vi "configure.vi"(8 "error in (no error)":errorcluster, 9 "Value":i32, 10 "ILC":refnum<class "ILC.lvclass">, 11 "ConfigureILCSSRStrategy in":refnum<class "ConfigureILCSSRStrategy.lvclass">) -> (0 "error out":errorcluster, 3 "ConfigureILCSSRStrategy out":refnum<class "ConfigureILCSSRStrategy.lvclass">)   [LabVIEW 2015, in "ConfigureILCSSRStrategy.lvclass"]
uses:
  ConfigureILCSSRStrategy.lvclass
  <userlib>/Common/ilc/ILC/ILC.lvclass
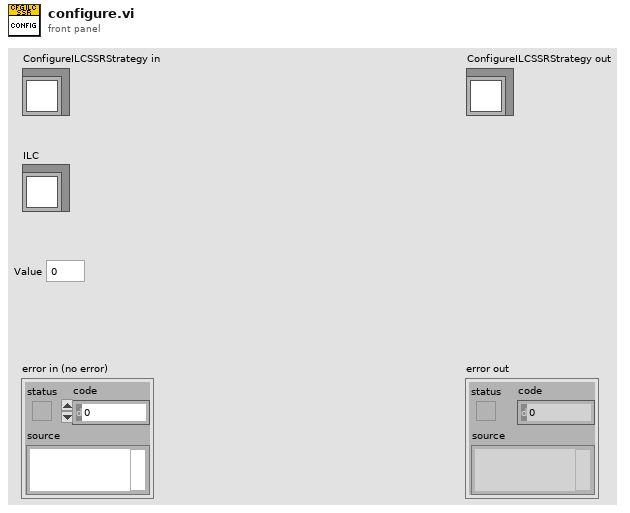
[diagram p1: front panel]
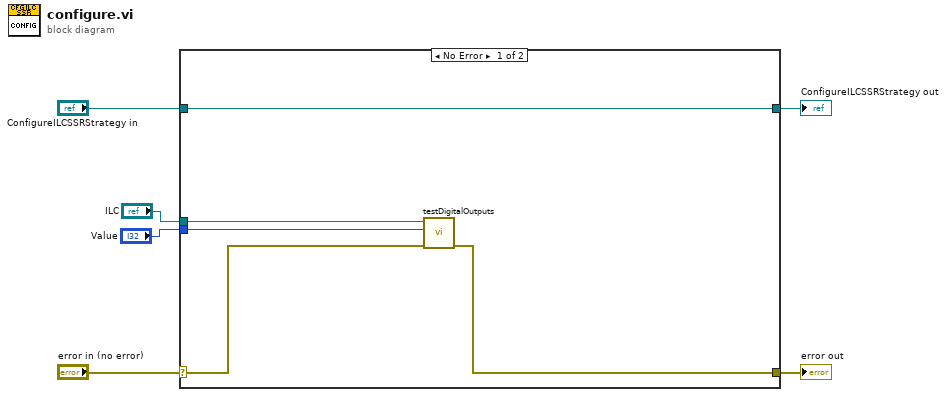
[diagram p0: block diagram]
diagram:
  n1 = case shown="No Error" "error in (no error)" {
    selector: "error in (no error)" -> [w7 w13]
    tunnel: [w8 w13] -> w5
    tunnel: [w11 w12] -> w3
    tunnel: "ConfigureILCSSRStrategy in" -> [w11 w12]
    tunnel: "ILC" -> [w10 _]
    tunnel: "Value" -> [w9 _]
    frame No Error {
      n2 = call <userlib>:"testDigitalOutputs.vi"("error in (no error)"=w7, "Digital Output Value"=w9, "ILC in"=w10) -> ("error out"=w8:errorcluster)  [unwired: 7 in, 1 out]
    }
    frame Error {
    }
  }
  "error out" <- w5
  "ConfigureILCSSRStrategy out" <- w3
